vi "Start.vi"(8 "error in (no error)":errorcluster, 11 "Sequence in":refnum<class "Sequence.lvclass">) -> (0 "error out":errorcluster, 3 "Sequence out":refnum<class "Sequence.lvclass">)   [LabVIEW 2018, in "Sequence.lvclass"]
doc: "compute # sweeps for the whole test.\nReplace Motion step type with Patch when this is not a motion test, an original hand connection test.\nSend UI message Start."
uses:
  Sequence.lvclass
  Support/MessageAPI/UIMessage.ctl
  Sequence.lvclass/Sequence.ctl
  SendMessage/SendMessage.lvclass
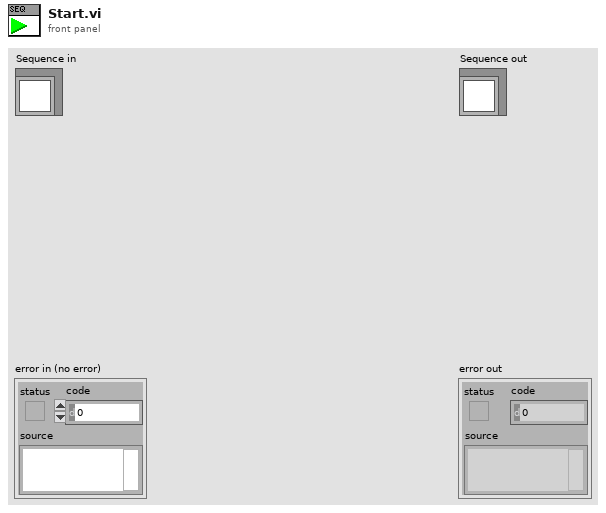
[diagram p1: front panel]
types:
  T1 = typedef "UIMessage.ctl" = cluster{"EventCode":i32, "Numeric":dbl, "String":string, "Variant":variant}
  T2 = typedef "mWaveTestStep.ctl" = cluster{"StepType":T3, "RF In/Out":T4, "Module/Raster":i32, "Polarization":T5, "AO-64 Array":dbl[], "Position":T6[]}
  T3 = typedef "TestStepTypes.ctl" = enum16{"MotionFF-M2", "Motion", "SweepTest", "RasterTest", "Finish", "64ModuleCfg"}
  T4 = typedef "RF Direction.ctl" = enum16{"Tx - RF In", "Rx - RF Out"}
  T5 = typedef "PolarizationSelect.ctl" = enum16{"Vertical", "Horizontal"}
  T6 = typedef "singleAxisMoveDef.ctl" = cluster{"mmWave Axis":T7, "eng. value":dbl}
  T7 = typedef "mmWaveAxis.ctl" = string
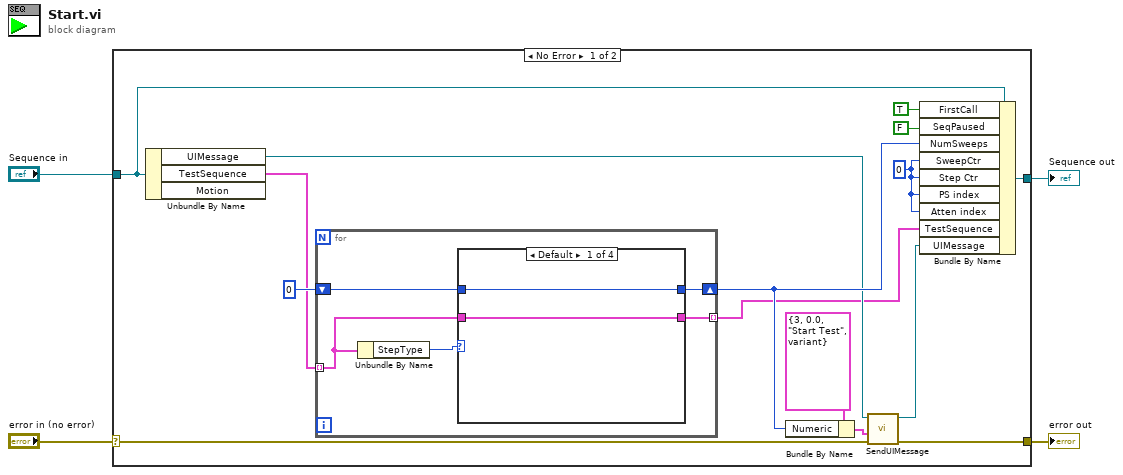
[diagram p0: block diagram]
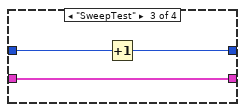
[diagram p3: hidden frame]
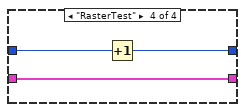
[diagram p4: hidden frame]
diagram:
  n1 = case shown="No Error" "error in (no error)" {
    selector: "error in (no error)" -> [w16 w36]
    tunnel: [w15 w36] -> w3
    tunnel: [w19 w35] -> w1
    tunnel: "Sequence in" -> [w18 w35]
    frame No Error {
      w10 = 0 ("Execution.Step Ctr")
      n2 = Unbundle By Name(w18) -> ("UIMessage"=w8:refnum<class "SendMessage.lvclass">, "TestSequence"=w5:T2[])  [unwired: 1 out]
      n3 = for {
        tunnel: w5 -> [w21] mode=indexing
        shift-right: [w23] -> w12
        shift-left: 0 -> [w22]
        tunnel: [w20] -> w6 mode=indexing
        n4 = Unbundle By Name(w21) -> ("StepType"=w24:T3)
        n5 = case shown="Default" w24 {
          tunnel: [w26 w28 w29 w33] -> w23
          tunnel: w22 -> [w26 w28 w30 w34]
          tunnel: w21 -> [w25 w27 w31 w32]
          tunnel: [w25 w27 w31 w32] -> w20
          frame Default {
          }
          frame "Motion" {
          }
          frame "SweepTest" {
            n6 = Increment(x=w30) -> (x+1=w29:i32)
          }
          frame "RasterTest" {
            n7 = Increment(x=w34) -> (x+1=w33:i32)
          }
        }
      }
      n8 = Bundle By Name(cluster=T1 {"EventCode"=3, "Numeric"=0.0, "String"="Start Test", "Variant"=variant} ("UIMsg"), "Numeric"=w12) -> (w14:T1)
      n9 = call-dynamic "SendUIMessage.vi"("error in (no error)"=w16, "UIMsg"=w14, "SendMessage in"=w8) -> ("error out"=w15:errorcluster, "SendMessage out"=w7:refnum<class "SendMessage.lvclass">)  [unwired: 7 in]
      n10 = Bundle By Name(cluster=w18, "FirstCall"=TRUE ("RF In/Out.FirstCall"), "SeqPaused"=FALSE, "NumSweeps"=w12, "SweepCtr"=w10, "Step Ctr"=w10, "PS index"=w10, "Atten index"=w10, "TestSequence"=w6, "UIMessage"=w7) -> (w19:refnum<class "Sequence.lvclass">)
    }
    frame Error {
    }
  }
  "error out" <- w3
  "Sequence out" <- w1
